vi "SoftSafety.vi"(4 "PositionData Translation":T1, 5 "PositionData Rotation":T1, 6 "AppliedTorqueRotation":dbl, 7 "AppliedForceTranslation":dbl) -> (3 "SoftSafety":bool)   [LabVIEW 2019]
uses:
  TypeDefs/PositionDataControl.ctl
panel:
  out "VelocityWithinBounds":bool
  out "PositionWithinBounds":bool
  out "TorqueWithinBounds":bool
  out "ForceWithinBounds":bool
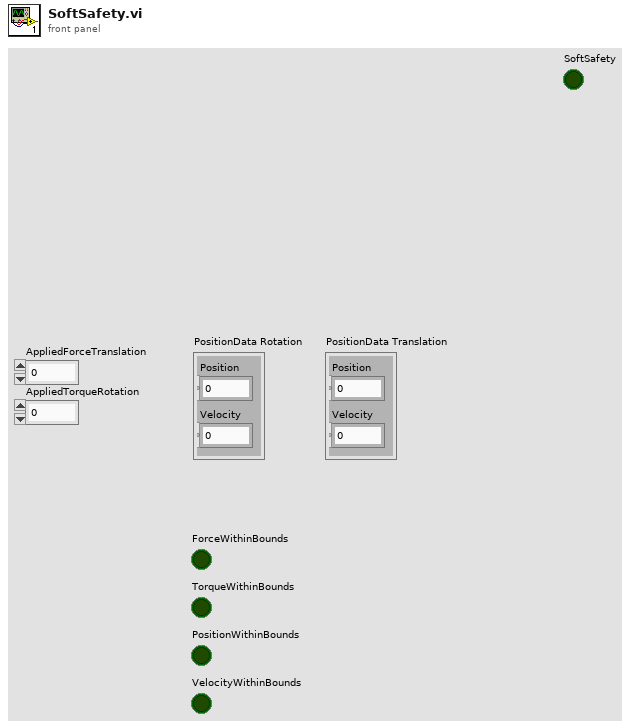
[diagram p1: front panel]
types:
  T1 = typedef "PositionDataControl.ctl" = cluster{"Position":dbl, "Velocity":dbl}
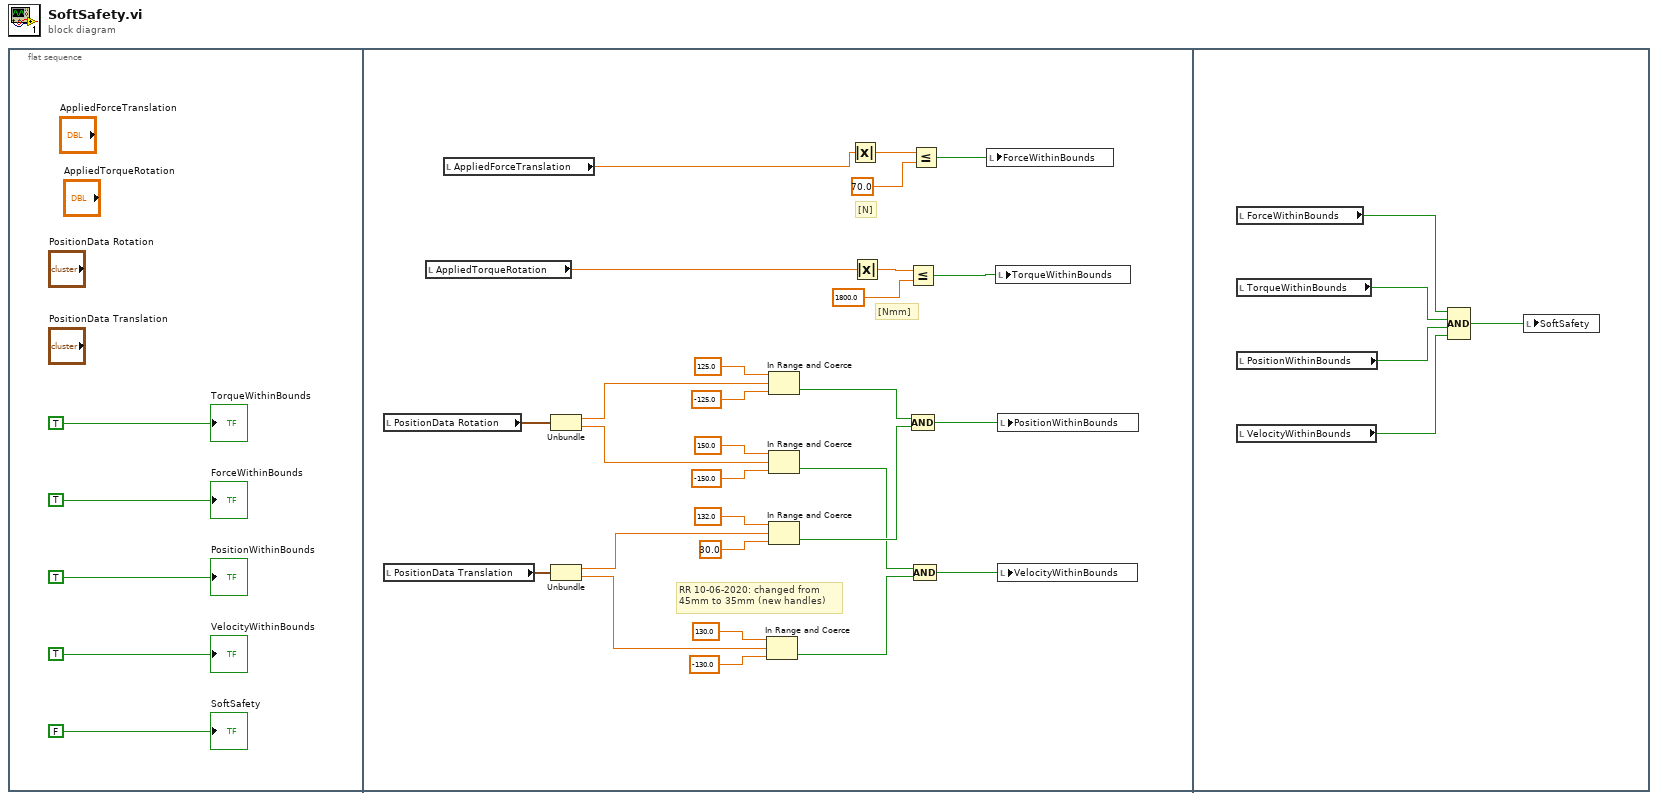
[diagram p0: block diagram]
diagram:
  n1 = flat-sequence {
    frame #0 {
      "TorqueWithinBounds" <- TRUE
      "ForceWithinBounds" <- TRUE
      "SoftSafety" <- FALSE
      "PositionWithinBounds" <- TRUE
      "VelocityWithinBounds" <- TRUE
    }
    frame #1 {
      # "[Nmm]"
      # "[N]"
      # "RR 10-06-2020: changed from\n45mm to 35mm (new handles)"
      n2 = local read "PositionData Rotation"() -> (w33:T1)
      n3 = local read "PositionData Translation"() -> (w18:T1)
      n4 = local read "AppliedTorqueRotation"() -> (w6:dbl)
      n5 = local read "AppliedForceTranslation"() -> (w7:dbl)
      n6 = Unbundle(w33) -> ("Position"=w32:dbl, "Velocity"=w27:dbl)
      n7 = Unbundle(w18) -> ("Position"=w19:dbl, "Velocity"=w24:dbl)
      n8 = In Range and Coerce(upper limit=130.0, x=w24, lower limit=-130.0) -> (In Range?=w14:bool)  [unwired: 1 out]
      n9 = In Range and Coerce(upper limit=125.0, x=w32, lower limit=-125.0) -> (In Range?=w26:bool)  [unwired: 1 out]
      n10 = In Range and Coerce(upper limit=150.0, x=w27, lower limit=-150.0) -> (In Range?=w15:bool)  [unwired: 1 out]
      n11 = In Range and Coerce(upper limit=132.0, x=w19, lower limit=30.0) -> (In Range?=w17:bool)  [unwired: 1 out]
      n12 = Absolute Value(x=w7) -> (abs(x)=w11:dbl)
      n13 = Absolute Value(x=w6) -> (abs(x)=w8:dbl)
      n14 = Less Or Equal?(x=w8, y=1800.0) -> (x <= y?=w10:bool)
      n15 = Less Or Equal?(x=w11, y=70.0) -> (x <= y?=w12:bool)
      n16 = Compound Arithmetic op=AND(w26, w17) -> (w25:bool)
      n17 = Compound Arithmetic op=AND(w15, w14) -> (w16:bool)
      n18 = local write "ForceWithinBounds"(w12) -> ()
      n19 = local write "TorqueWithinBounds"(w10) -> ()
      n20 = local write "PositionWithinBounds"(w25) -> ()
      n21 = local write "VelocityWithinBounds"(w16) -> ()
    }
    frame #2 {
      n22 = local read "ForceWithinBounds"() -> (w37:bool)
      n23 = local read "TorqueWithinBounds"() -> (w36:bool)
      n24 = local read "PositionWithinBounds"() -> (w35:bool)
      n25 = local read "VelocityWithinBounds"() -> (w34:bool)
      n26 = Compound Arithmetic op=AND(w37, w36, w35, w34) -> (w38:bool)
      n27 = local write "SoftSafety"(w38) -> ()
    }
  }
